vi "Simple_switch.vi"() -> ()   [LabVIEW 2023]
uses:
  LabVIEW/Lab4_235/Serial - Settings.ctl
  <vilib>/Instr/_visa.llb/VISA Configure Serial Port (Instr).vi
panel:
  in  "stop":bool
  in  "Switch":bool
  out "Read Buffer":string
  in  "Serial Settings":T1={"baud rate"=115200, "data bits"=8, "parity"=enum."None", "stop bits"=10, "flow control"=0} {"flow control" items=["None"=0, "XON/XOFF"=1, "RTS/CTS"=2, "DTR/DSR"=4]; "stop bits" items=["1.0"=10, "1.5"=15, "2.0"=20]; "data bits" min=5 max=8 step=1; "baud rate" items=["75"=75, "110"=110, "134"=134, "150"=150, "300"=300, "600"=600, "1200"=1200, "1800"=1800, "2400"=2400, "4800"=4800, "7200"=7200, "9600"=9600, "14400"=14400, "19200"=19200, "28800"=28800, "38400"=38400, "56000"=56000, "57600"=57600, "115200"=115200, "128000"=128000, "230400"=230400]}
  in  "VISA resource name":refnum<visa-resource-name>
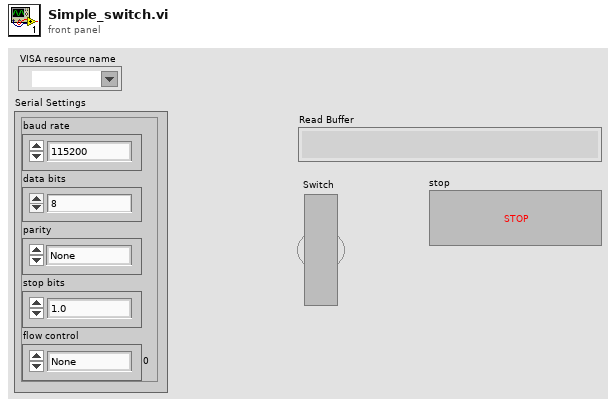
[diagram p1: front panel]
types:
  T1 = typedef "Serial - Settings.ctl" = cluster{"baud rate":u32, "data bits":u16, "parity":enum16{"None", "Odd", "Even", "Mark", "Space"}, "stop bits":u16, "flow control":u16}
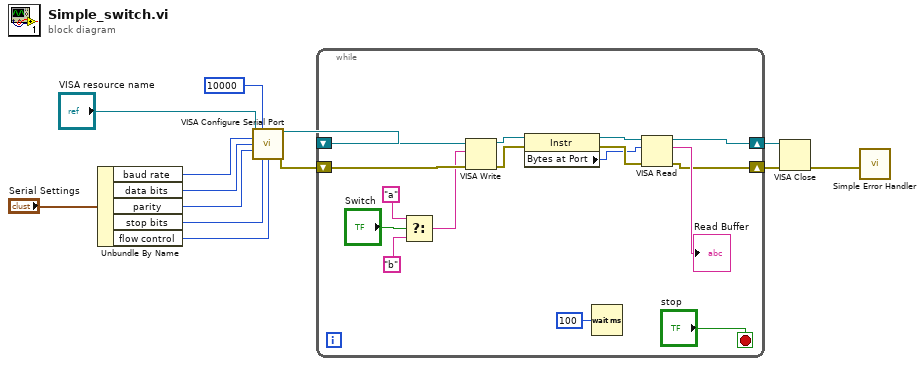
[diagram p0: block diagram]
diagram:
  n1 = Unbundle By Name("Serial Settings") -> ("baud rate"=w11:u32, "data bits"=w10:u16, "parity"=w9:enum16{"None", "Odd", "Even", "Mark", "Space"}, "stop bits"=w8:u16, "flow control"=w7:u16)
  n2 = call-poly "VISA Configure Serial Port"("VISA resource name"="VISA resource name", "timeout (10sec)"=u32 10000, "baud rate (9600)"=w11, "data bits (8)"=w10, "parity (0:none)"=w9, "stop bits (10: 1 bit)"=w8, "flow control (0:none)"=w7) -> ("VISA resource name out"=w6:refnum<visa-resource-name>, "error out"=w4:errorcluster)  [unwired: 7 in]
  n3 = while {
    shift-right: [w27] -> w5
    shift-left: w6 -> [w29]
    shift-right: [w21] -> w3
    shift-left: w4 -> [w22]
    stop <- "stop" stop-if-true
    n4 = Select(t="a", s="Switch", f="b") -> (s? t:f=w16:string)
    n5 = VISA Write(VISA resource name=w29, write buffer=w16, error in (no error)=w22) -> (VISA resource name out=w26:refnum<visa-resource-name>, error out=w24:errorcluster)  [unwired: 1 out]
    n6 = property on="Property Node" class="Instr"(reference=w26, error in=w24) -> (reference out=w25:refnum<visa-resource-name>, error out=w23:errorcluster, "Bytes at Port"=w20:u32)
    n7 = Wait (ms)(milliseconds to wait=u32 100) -> ()  [unwired: 1 out]
    n8 = VISA Read(VISA resource name=w25, byte count=w20, error in (no error)=w23) -> (VISA resource name out=w27:refnum<visa-resource-name>, read buffer=→"Read Buffer":string, error out=w21:errorcluster)  [unwired: 1 out]
  }
  n9 = VISA Close(VISA resource name=w5, error in (no error)=w3) -> (error out=w1:errorcluster)
  n10 = call <vilib>:"Simple Error Handler.vi"("error in (no error)"=w1) -> ()  [unwired: 4 in, 5 out]
